vi "CRYSet Get Message VI Name Front Panel.vi"(11 "Vi Ref":refnum<vi>) -> ()   [LabVIEW 2013]
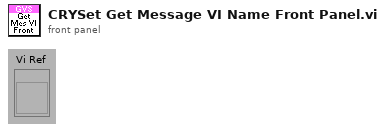
[diagram p1: front panel]
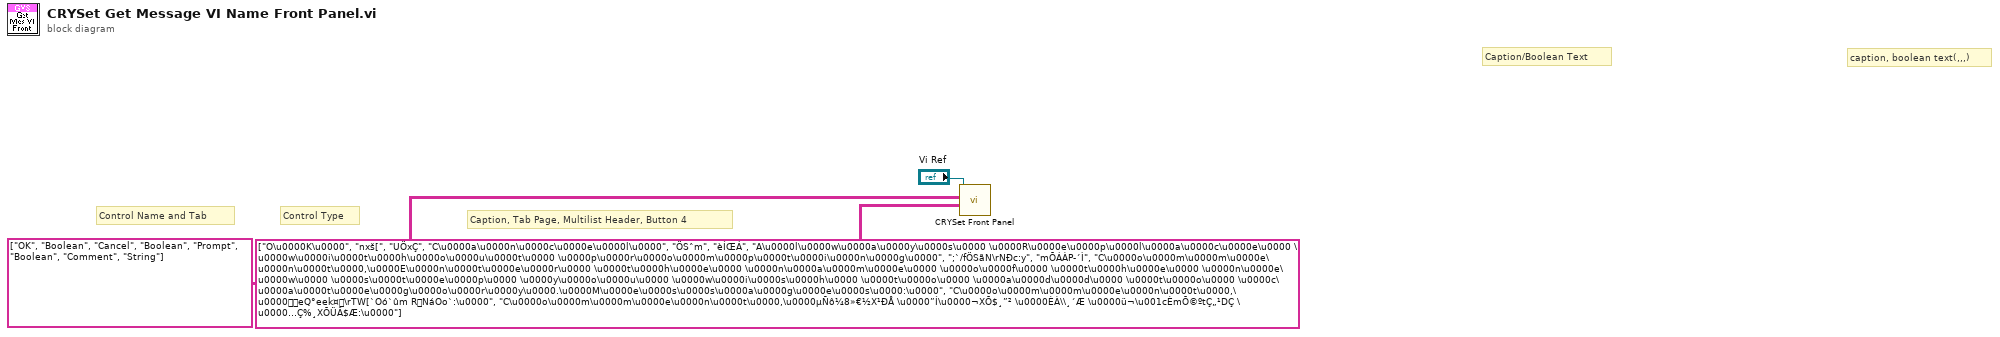
[diagram p0: block diagram]
diagram:
  # "Caption, Tab Page, Multilist Header, Button 4"
  # "Control Type"
  # "Control Name and Tab"
  # "caption, boolean text(,,,)"
  # "Caption/Boolean Text"
  n1 = call "CRYSet Front Panel.vi"("Caption(Boolean Text)"=string[][] [["O\u0000K\u0000", "nxš[", "UÖxÇ"], ["C\u0000a\u0000n\u0000c\u0000e\u0000l\u0000", "ÖSˆm", "èÍŒÁ"], ["A\u0000l\u0000w\u0000a\u0000y\u0000s\u0000 \u0000R\u0000e\u0000p\u0000l\u0000a\u0000c\u0000e\u0000 \u0000w\u0000i\u0000t\u0000h\u0000o\u0000u\u0000t\u0000 \u0000p\u0000r\u0000o\u0000m\u0000p\u0000t\u0000i\u0000n\u0000g\u0000", ";`/fÖSãN\rNÐc:y", "mÕÁÀP­´Ì"], ["C\u0000o\u0000m\u0000m\u0000e\u0000n\u0000t\u0000,\u0000E\u0000n\u0000t\u0000e\u0000r\u0000 \u0000t\u0000h\u0000e\u0000 \u0000n\u0000a\u0000m\u0000e\u0000 \u0000o\u0000f\u0000 \u0000t\u0000h\u0000e\u0000 \u0000n\u0000e\u0000w\u0000 \u0000s\u0000t\u0000e\u0000p\u0000 \u0000y\u0000o\u0000u\u0000 \u0000w\u0000i\u0000s\u0000h\u0000 \u0000t\u0000o\u0000 \u0000a\u0000d\u0000d\u0000 \u0000t\u0000o\u0000 \u0000c\u0000a\u0000t\u0000e\u0000g\u0000o\u0000r\u0000y\u0000.\u0000M\u0000e\u0000s\u0000s\u0000a\u0000g\u0000e\u0000s\u0000:\u0000", "C\u0000o\u0000m\u0000m\u0000e\u0000n\u0000t\u0000,\u0000eQ°eek¤\rTW[`Oó`ûm RNáOo`:\u0000", "C\u0000o\u0000m\u0000m\u0000e\u0000n\u0000t\u0000,\u0000µÑô¼8»€½X¹ÐÅ \u0000”Í\u0000¬XÕ$¸”² \u0000ÈÀ\\¸´Æ \u0000ü¬\u001cÈmÕ©ºtÇ„¹DÇ \u0000…Ç%¸XÕÜÂ$Æ:\u0000"]], "Control ID and Type(Label Name, Type)"=string[][] [["OK", "Boolean"], ["Cancel", "Boolean"], ["Prompt", "Boolean"], ["Comment", "String"]], "Vi Ref"="Vi Ref") -> ()  [unwired: 9 in]
